vi "Email Shifter.vi"   [LabVIEW 2013]
uses:
  <vilib>/smtpClient/Set Message Text.vi
  <vilib>/smtpClient/LabVIEWSMTPClient.lvlib
types:
  T1 = typedef "LabVIEWSMTPClient.lvlib/SmtpClientHandle.ctl" = refnum<k1>
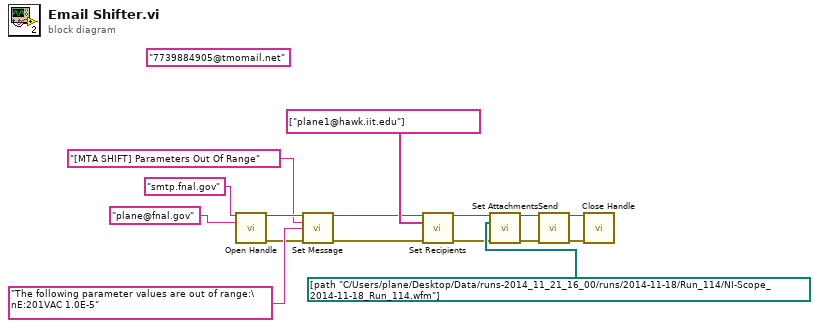
[diagram p0: block diagram]
diagram:
  (unwired) "7739884905@tmomail.net" ("Recipients")
  n1 = call <vilib>:"Open Handle.vi"("server address"="smtp.fnal.gov", "from"="plane@fnal.gov") -> ("handle out"=w14:T1, "error out"=w9:errorcluster)  [unwired: 12 in]
  n2 = call-poly <vilib>:"Set Message.vi"("handle in"=w14, "subject"="[MTA SHIFT] Parameters Out Of Range" ("Subject"), "plain text message"="The following parameter values are out of range:\nE:201VAC 1.0E-5" ("Message"), "error in (no error)"=w9) -> ("handle out"=w10:T1, "error out"=w8:errorcluster)  [unwired: 10 in]
  n3 = call <vilib>:"Set Recipients.vi"("handle in"=w10, "to"=string[] ["plane1@hawk.iit.edu"], "error in (no error)"=w8) -> ("handle out"=w7:T1, "error out"=w5:errorcluster)  [unwired: 11 in]
  n4 = call <vilib>:"Set Attachments.vi"("handle in"=w7, "attachments"=path[] [path "C:/Users/plane/Desktop/Data/runs-2014_11_21_16_00/runs/2014-11-18/Run_114/NI-Scope_2014-11-18_Run_114.wfm"], "error in (no error)"=w5) -> ("handle out"=w4:T1, "error out"=w3:errorcluster)  [unwired: 11 in]
  n5 = call <vilib>:"Send.vi"("handle in"=w4, "error in (no error)"=w3) -> ("handle out"=w2:T1, "error out"=w1:errorcluster)  [unwired: 11 in, 1 out]
  n6 = call <vilib>:"Close Handle.vi"("handle in"=w2, "error in (no error)"=w1) -> ()  [unwired: 12 in, 2 out]
